vi "parse_accel_roslv.vi"(4 "error in":errorcluster, 7 "msg in":string) -> (0 "error out":errorcluster, 2 "Accel":T1, 3 "msg out":string)   [LabVIEW 2014]
doc: "Parses a message into an acceleration"
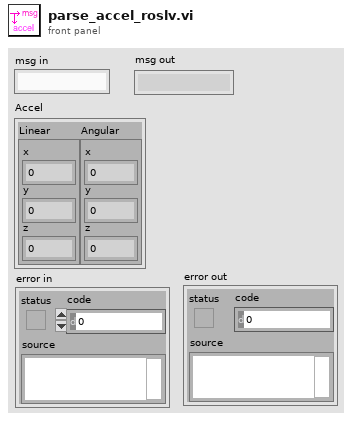
[diagram p1: front panel]
types:
  T1 = cluster{"Linear":cluster{"x":dbl, "y":dbl, "z":dbl}, "Angular":cluster{"x":dbl, "y":dbl, "z":dbl}}
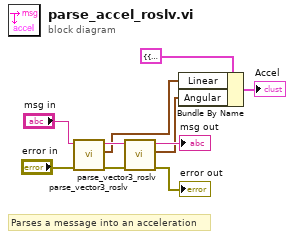
[diagram p0: block diagram]
diagram:
  # "Parses a message into an acceleration"
  n1 = call "parse_vector3_roslv.vi"("error in"="error in", "msg in"="msg in") -> ("error out"=w7:errorcluster, "Vector3"=w3:cluster{"x":dbl, "y":dbl, "z":dbl}, "msg out"=w9:string)  [unwired: 3 in]
  n2 = call "parse_vector3_roslv.vi"("error in"=w7, "msg in"=w9) -> ("error out"=→"error out":errorcluster, "Vector3"=w2:cluster{"x":dbl, "y":dbl, "z":dbl}, "msg out"=→"msg out":string)  [unwired: 3 in]
  n3 = Bundle By Name(cluster=T1 {"Linear"={"x"=0.0, "y"=0.0, "z"=0.0}, "Angular"={"x"=0.0, "y"=0.0, "z"=0.0}} ("input cluster"), "Linear"=w3, "Angular"=w2) -> (→"Accel":T1)
